vi "Setup subWorker - TCP Client.vi"(8 "error in":errorcluster, 11 "Head Worker in":refnum<class "Head Worker.lvclass">) -> (0 "error out":errorcluster, 3 "Head Worker out":refnum<class "Head Worker.lvclass">)   [LabVIEW 2017, in "Head Worker.lvclass"]
doc: "This VI sets up the framework parameters of a statically-linked subWorker."
uses:
  Head Worker.lvclass
  Head Worker.lvclass/Head Worker.ctl
  TCP Client/TCP Client/TCP Client.lvclass
  C:/Program Files (x86)/National Instruments/LabVIEW 2017/vi.lib/addons/_Workers/Library/Classes/Worker/Worker.lvclass
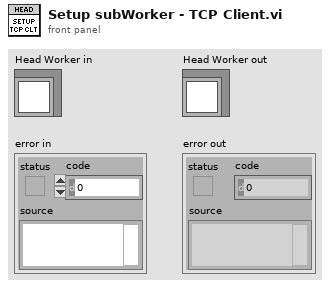
[diagram p1: front panel]
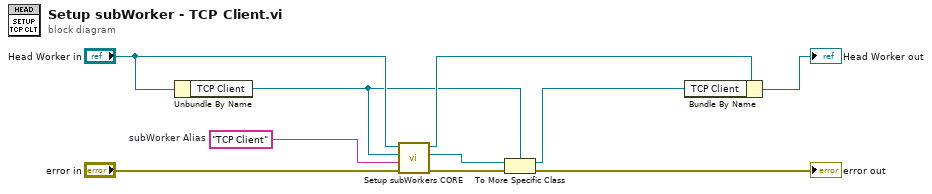
[diagram p0: block diagram]
diagram:
  w6 = "TCP Client"  # subWorker Alias
  n1 = Unbundle By Name("Head Worker in") -> ("TCP Client"=w3:refnum<class "TCP Client.lvclass">)
  n2 = call-dynamic "Setup subWorkers CORE.vi"("error in"="error in", "subWorker Alias"=w6, "subWorker"=w3, "Worker"="Head Worker in") -> ("error out"=w5:errorcluster, "subWorker out"=w1:refnum<class "Worker.lvclass">, "Worker out"=w8:refnum<class "Head Worker.lvclass">)  [unwired: 5 in]
  n3 = To More Specific Class(target class=w3, reference=w1, error in=w5) -> (specific class reference=w2:refnum<class "TCP Client.lvclass">, error out=→"error out":errorcluster)
  n4 = Bundle By Name(cluster=w8, "TCP Client"=w2) -> (→"Head Worker out":refnum<class "Head Worker.lvclass">)
